vi "Get Selected Channel Settings.vi"(8 "error in (no error)":errorcluster, 11 "Refs":refnum<k24>[](array[refnum])) -> (0 "error out":errorcluster, 1 "Path":string[](array[string]), 2 "Name":string[](array[string]), 3 "IDs":u64[](array[numeric]))   [LabVIEW 2026, in "WebPage Addon System Explorer.lvlib"]
uses:
  WebPage Addon System Explorer.lvlib
  NationalInstruments.VeriStand.SystemStorage
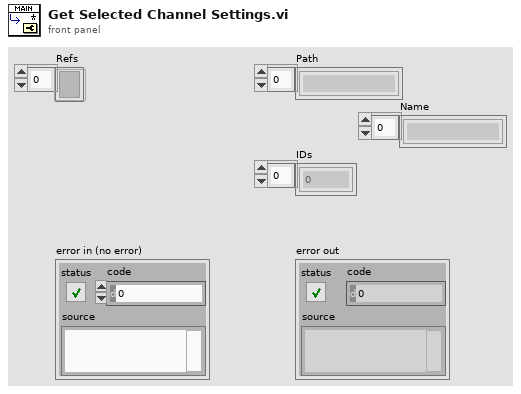
[diagram p1: front panel]
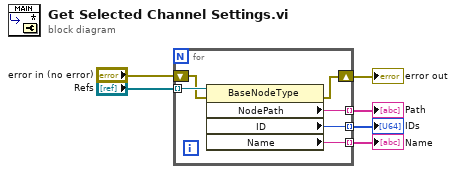
[diagram p0: block diagram]
diagram:
  n1 = for {
    tunnel: "Refs" -> [w12] mode=indexing
    tunnel: [w8] -> w3 mode=indexing
    tunnel: [w11] -> w4 mode=indexing
    shift-right: [w9] -> w6
    shift-left: "error in (no error)" -> [w10]
    tunnel: [w7] -> w1 mode=indexing
    n2 = property class="BaseNodeType"(reference=w12, error in=w10) -> (error out=w9:errorcluster, "NodePath"=w8:string, "ID"=w11:u64, "Name"=w7:string)  [unwired: 1 out]
  }
  "error out" <- w6
  "IDs" <- w4
  "Path" <- w3
  "Name" <- w1
